vi "Create Plugin.vi"(7 "Configuration Entry":string, 8 "error in (no error)":errorcluster, 11 "Configuration Parameters":string[](array[string])) -> (0 "error out":errorcluster, 2 "Logic Entry":T1, 3 "Configuration Entry":T1)   [LabVIEW 2021, in "Python Orchestration.lvlib"]
uses:
  Python Orchestration.lvlib
  Typedef/Scripted Line.ctl
  CIFCore/Common/Typedef/Errors.ctl
  <vilib>/CIF Foundation/CIF Utilities/Errors/Append Error Location.vi
  CIFCore/Common/CIFCoreCommon.lvlib
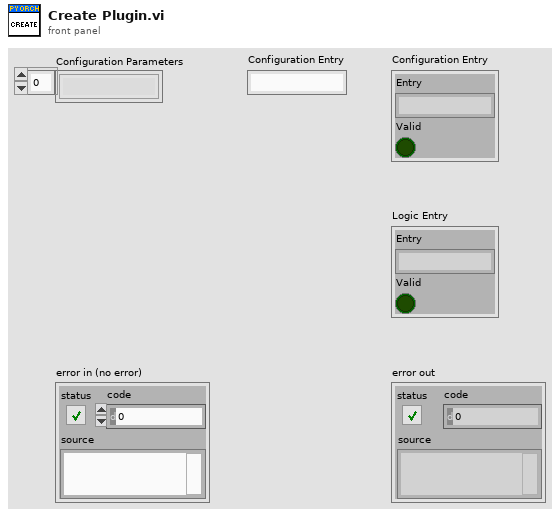
[diagram p1: front panel]
types:
  T1 = typedef "Python Orchestration.lvlib/Scripted Line.ctl" = cluster{"Entry":string, "Valid":bool}
  T2 = typedef "CIFCoreCommon.lvlib/Errors.ctl" = enum16{"Invalid Clock ID", "Long Sleep", "gRPC Server Not Found", "Config Parse", "Timestamp Wrap", "Delayed Execution", "Duplicate Channel", "Missing Channel", "Incorrect Type", "Flatten Error", "Unflatten Data", "Unique Name", "Plugin Not Found", "Plugin Type Not Found", "Plugin Version Not Found", "Manager Not Found", "Numerical Issue", "Time Jump", "Clock ID Match", "Channel Length", "Plugin Connection", "gRPC Server Connection", "PPL Name Match", "Build", "Config Log Parse", "Plugin Load", "UI Subpanel Load"}
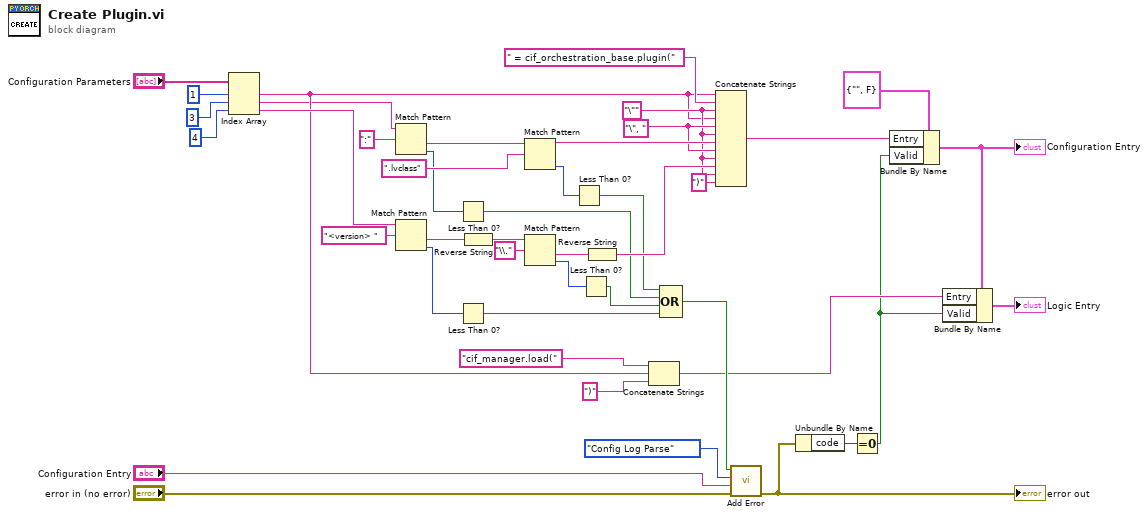
[diagram p0: block diagram]
diagram:
  w35 = "\", "
  w26 = "\""
  n1 = Index Array(array="Configuration Parameters", index #1=1 ("index"), index #2=3 ("index"), index #3=4 ("index")) -> (element #1=w24:string, element #2=w19:string, element #3=w33:string)
  n2 = Match Pattern(string=w19, regular expression=":") -> (after substring=w38:string, offset past match=w23:i32)  [unwired: 1 in, 2 out]
  n3 = Match Pattern(string=w33, regular expression="<version> ") -> (after substring=w31:string, offset past match=w21:i32)  [unwired: 1 in, 2 out]
  n4 = Less Than 0?(x=w23) -> (x < 0?=w16:bool)
  n5 = Less Than 0?(x=w21) -> (x < 0?=w18:bool)
  n6 = Reverse String(1:w31) -> (0:w30:string)
  n7 = Match Pattern(string=w38, regular expression=".lvclass") -> (before substring=w36:string, offset past match=w22:i32)  [unwired: 1 in, 2 out]
  n8 = Match Pattern(string=w30, regular expression="\\.") -> (after substring=w28:string, offset past match=w20:i32)  [unwired: 1 in, 2 out]
  n9 = Less Than 0?(x=w22) -> (x < 0?=w15:bool)
  n10 = Less Than 0?(x=w20) -> (x < 0?=w17:bool)
  n11 = Reverse String(1:w28) -> (0:w27:string)
  n12 = Concatenate Strings("cif_manager.load(", w24, ")" ("string")) -> (w7:string)
  n13 = Compound Arithmetic op=OR(w15, w16, w17, w18) -> (w14:bool)
  n14 = Concatenate Strings(w24, " = cif_orchestration_base.plugin(", w26, w24, w35, w26, w36, w35, w26, w27, w26, ")" ("string")) -> (w10:string)
  n15 = call "Add Error.vi"("error in (no error)"="error in (no error)", "String to Append"="Configuration Entry", "Error"=Errors."Config Log Parse", "Insert Error"=w14) -> ("error out"=w9:errorcluster)  [unwired: 7 in]
  "error out" <- w9
  n16 = Unbundle By Name(w9) -> ("code"=w8:i32)
  n17 = Equal To 0?(x=w8) -> (x = 0?=w6:bool)
  n18 = Bundle By Name(cluster=T1 {"Entry"="", "Valid"=FALSE} ("Logic Entry"), "Entry"=w10, "Valid"=w6) -> (w3:T1)
  "Configuration Entry" <- w3
  n19 = Bundle By Name(cluster=w3, "Entry"=w7, "Valid"=w6) -> (→"Logic Entry":T1)
